vi "Str.Str to Float, Check if is Number.vi"(11 "Value In":string) -> (2 "Num Out":dbl, 3 "Value Out":string, 5 "Is Num":bool)   [LabVIEW 2018]
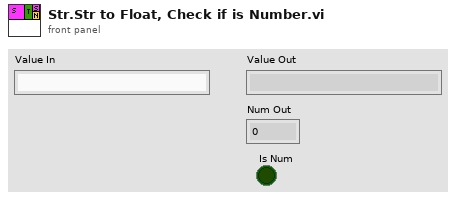
[diagram p1: front panel]
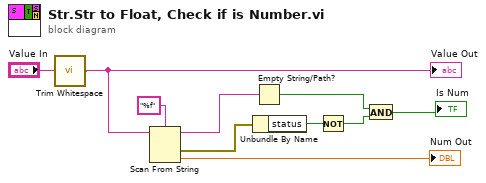
[diagram p0: block diagram]
diagram:
  n1 = call <vilib>:"Trim Whitespace.vi"("string"="Value In") -> ("trimmed string"=w1:string)  [unwired: 1 in]
  "Value Out" <- w1
  n2 = Scan From String(format string="%f", input string=w1) -> (remaining string=w7:string, error out=w8:errorcluster, output 1=→"Num Out":dbl)  [unwired: 3 in, 1 out]
  n3 = Unbundle By Name(w8) -> ("status"=w6:bool)
  n4 = Empty String/Path?(string/path=w7) -> (empty?=w4:bool)
  n5 = Not(x=w6) -> (.not. x?=w5:bool)
  n6 = And(x=w4, y=w5) -> (x .and. y?=→"Is Num":bool)
